vi "Update Class and Library Names.vi"(7 "Overlay Icon":refnum<class "Icon.lvclass">, 8 "error in (no error)":errorcluster, 9 "Type ID":string="Test", 10 "New Name":string="Test", 11 "Project Path":path) -> (0 "error out":errorcluster)   [LabVIEW 2020, in "ADAS_IO_Template_MDO.lvclass"]
uses:
  ADAS_IO_Template_MDO.lvclass
  <vilib>/LabVIEW Icon API/lv_icon/Classes/Icon/Icon.lvclass
  ADAS_IO_Template_MDO.lvclass/ADAS_IO_Template_MDO.ctl
  <vilib>/Utility/EditLVLibs/Edit LVLibs.lvlib
  <vilib>/Utility/EditLVProj/Edit LVProj.lvlib
  <vilib>/LabVIEW Icon API/LabVIEW Icon API.lvlib
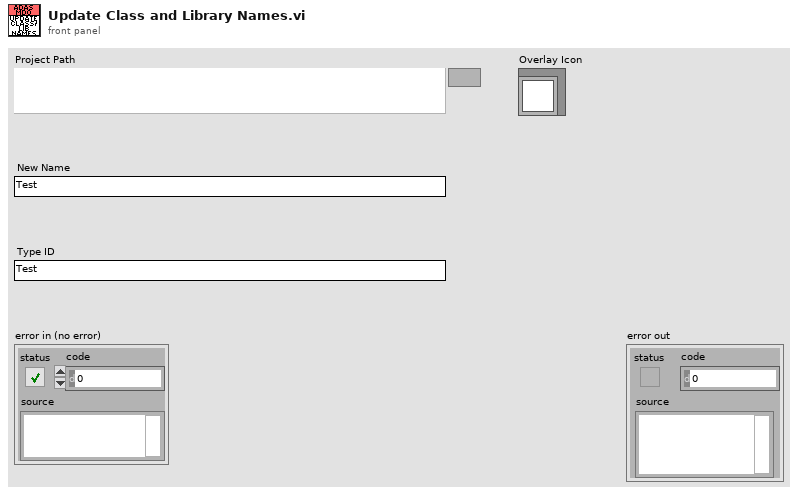
[diagram p1: front panel]
types:
  T1 = typedef "Edit LVProj.lvlib/Library And VI References.ctl" = cluster{"Target Reference":refnum<vi>, "VI References":refnum<vi>[], "Library References":refnum<vi>[]}
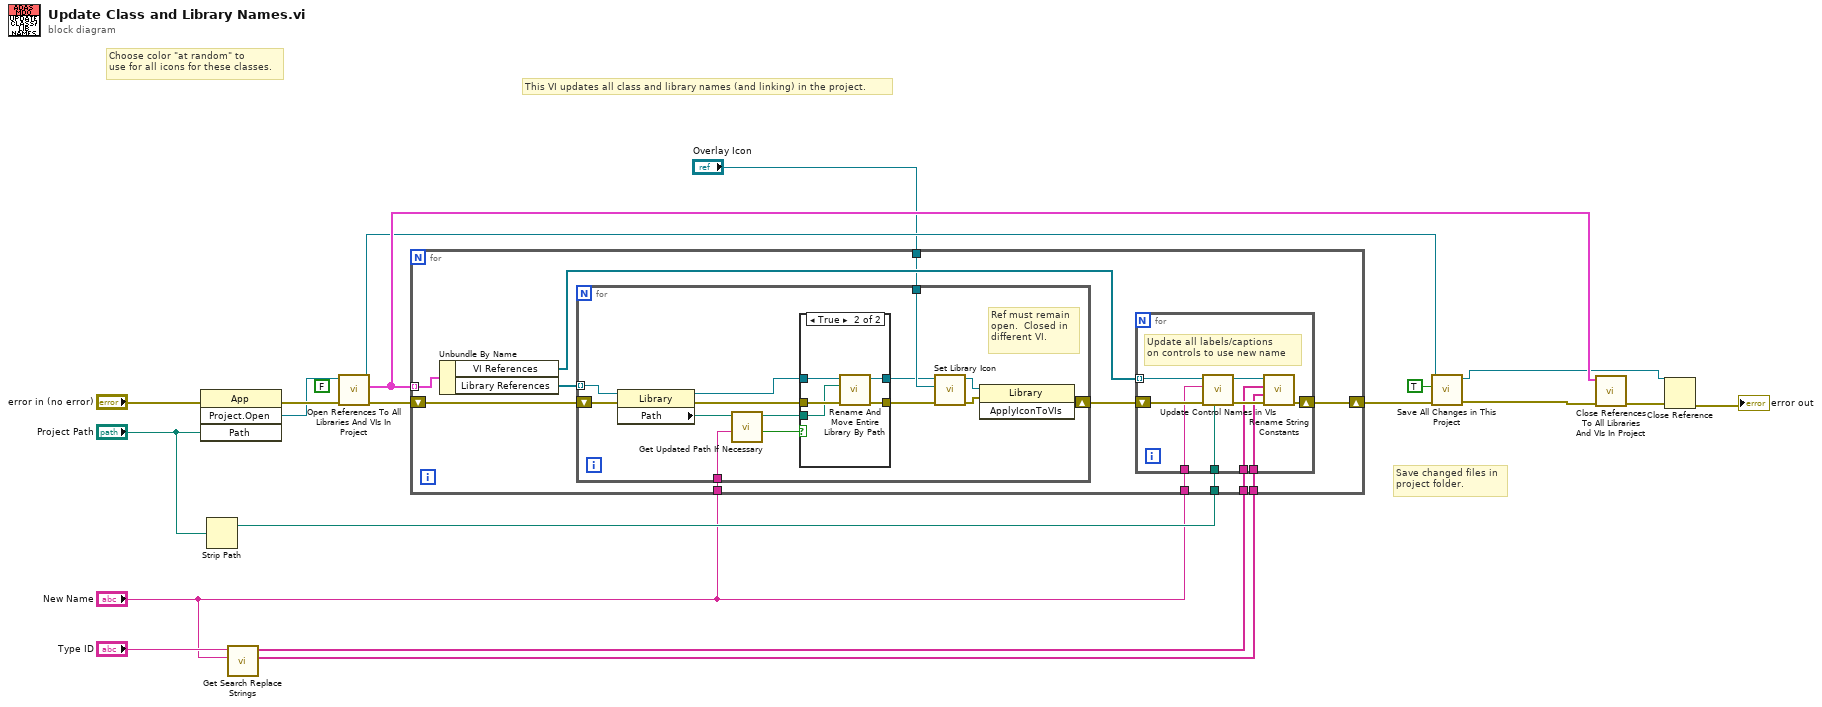
[diagram p0: block diagram]
diagram:
  (unwired) FALSE ("Exclude Dependencies? (T)")
  # "Save changed files in\nproject folder."
  # "Choose color \"at random\" to\nuse for all icons for these classes."
  # "This VI updates all class and library names (and linking) in the project."
  n1 = invoke class="App" method="Project.Open"(error in="error in (no error)", "Path"="Project Path") -> (error out=w18:errorcluster, "Project:Open"=w16:refnum<vi>)  [unwired: 2 in, 2 out]
  n2 = Strip Path(path="Project Path") -> (stripped path=w10:path)  [unwired: 1 out]
  n3 = call "Get Search Replace Strings.vi"("New Name"="New Name", "GUID"="Type ID") -> ("Replacement Strings"=w6:string[], "Search Strings"=w7:string[])  [unwired: 8 in]
  n4 = call <vilib>:"Open References To All Libraries And VIs In Project.vi"("error in (no error)"=w18, "Project in"=w16) -> ("error out"=w17:errorcluster, "VI and Library References"=w15:T1[], "Project out"=w14:refnum<vi>)  [unwired: 7 in]
  n5 = for {
    tunnel: w15 -> [w31] mode=indexing
    shift-right: [w25] -> w13
    shift-left: w17 -> [w30]
    tunnel: "New Name" -> [w28]
    tunnel: "New Name" -> [w24]
    tunnel: w10 -> [w23]
    tunnel: w7 -> [w22]
    tunnel: w6 -> [w21]
    tunnel: "Overlay Icon" -> [w20]
    n6 = Unbundle By Name(w31) -> ("VI References"=w27:refnum<vi>[], "Library References"=w29:refnum<vi>[])
    n7 = for {
      shift-right: [w41] -> w26
      shift-left: w30 -> [w54]
      tunnel: w29 -> [w53] mode=indexing
      tunnel: w28 -> [w51]
      tunnel: w20 -> [w46]
      # "Ref must remain\nopen.  Closed in\ndifferent VI."
      n8 = property class="Library"(reference=w53, error in=w54) -> (reference out=w47:refnum<vi>, error out=w50:errorcluster, "Path"=w52:path)
      n9 = call "Get Updated Path If Necessary.vi"("New Name"=w51, "Original Path"=w52) -> ("Update?"=w49:bool, "New Path"=w48:path)  [unwired: 8 in]
      n10 = case shown="True" w49 {
        tunnel: w47 -> [w55 w61]
        tunnel: w50 -> [w56 w60]
        tunnel: w48 -> [_ w59]
        tunnel: [w56 w58] -> w44
        tunnel: [w55 w57] -> w45
        frame False {
        }
        frame True {
          n11 = call <vilib>:"Rename And Move Entire Library By Path.vi"("error in (no error)"=w60, "New library path"=w59, "Library ref in"=w61) -> ("error out"=w58:errorcluster, "Library ref out"=w57:refnum<vi>)  [unwired: 7 in]
        }
      }
      n12 = call <vilib>:"Set Library Icon.vi"("error in (no error)"=w44, "Icon"=w46, "Library Refnum in"=w45) -> ("error out"=w42:errorcluster, "Library Refnum out"=w43:refnum<vi>)  [unwired: 7 in]
      n13 = invoke class="Library" method="ApplyIconToVIs"(reference=w43, error in=w42) -> (error out=w41:errorcluster)  [unwired: 1 in, 2 out]
    }
    n14 = for {
      tunnel: w27 -> [w38] mode=indexing
      shift-right: [w35] -> w25
      shift-left: w26 -> [w40]
      tunnel: w24 -> [w39]
      tunnel: w23 -> [w37]
      tunnel: w22 -> [w33]
      tunnel: w21 -> [w32]
      # "Update all labels/captions\non controls to use new name"
      n15 = call "Update Control Names in VIs.vi"("Build Folder"=w37, "error in (no error)"=w40, "New Name"=w39, "VI Reference"=w38) -> ("error out"=w36:errorcluster, "vi ref out"=w34:refnum<vi>)  [unwired: 6 in]
      n16 = call "Rename String Constants.vi"("error in (no error)"=w36, "Replace Strings"=w32, "Search Strings"=w33, "vi reference"=w34) -> ("error out"=w35:errorcluster)  [unwired: 6 in, 1 out]
    }
  }
  n17 = call "Save All Changes in This Project.vi"("error in (no error)"=w13, "Exclude Dependencies? (F)"=TRUE, "Project in"=w14) -> ("error out"=w4:errorcluster, "Project out"=w3:refnum<vi>)  [unwired: 7 in]
  n18 = call <vilib>:"Close References To All Libraries And VIs In Project.vi"("error in (no error)"=w4, "VI and Library References"=w15) -> ("error out"=w2:errorcluster)  [unwired: 9 in]
  n19 = Close Reference(reference=w3, error in (no error)=w2) -> (error out=→"error out":errorcluster)
